vi "roboRIO Set Pin Info.vi"(7 "Size":i32=30, 9 "Pin Info Array":T2, 11 "Display State In in":T1 caption="State") -> (1 "Data":bool[](array[boolean]), 3 "Display State In out":T1 caption="State")   [LabVIEW 2021]
uses:
  <vilib>/myRIO/Common/Instrument Driver Framework/Utilities/xctls/utilities/typedefs/myRIOXC Pin Info Array.ctl
  <vilib>/myRIO/Common/Instrument Driver Framework/Utilities/xctls/utilities/typedefs/myRIOXC Pin Info.ctl
  <vilib>/myRIO/Common/Instrument Driver Framework/Utilities/xctls/utilities/typedefs/roboRIO Bank Display State.ctl
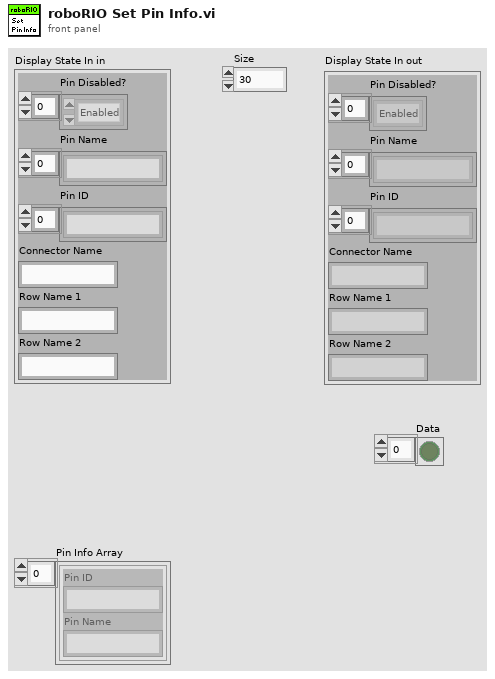
[diagram p1: front panel]
types:
  T1 = typedef "roboRIO Bank Display State.ctl" = cluster{"Pin Disabled?":enum8{"Enabled", "Disabled", "Disabled and Grayed Out"}[], "Pin Name":string[], "Pin ID":string[], "Connector Name":string, "Row Name 1":string, "Row Name 2":string}
  T2 = typedef "myRIOXC Pin Info Array.ctl" = T3[]
  T3 = typedef "myRIOXC Pin Info.ctl" = cluster{"Pin ID":string, "Pin Name":string}
  T4 = enum8{"Enabled", "Disabled", "Disabled and Grayed Out"}
  T5 = enum8{"Enabled", "Disabled", "Disabled and Grayed Out"}[]
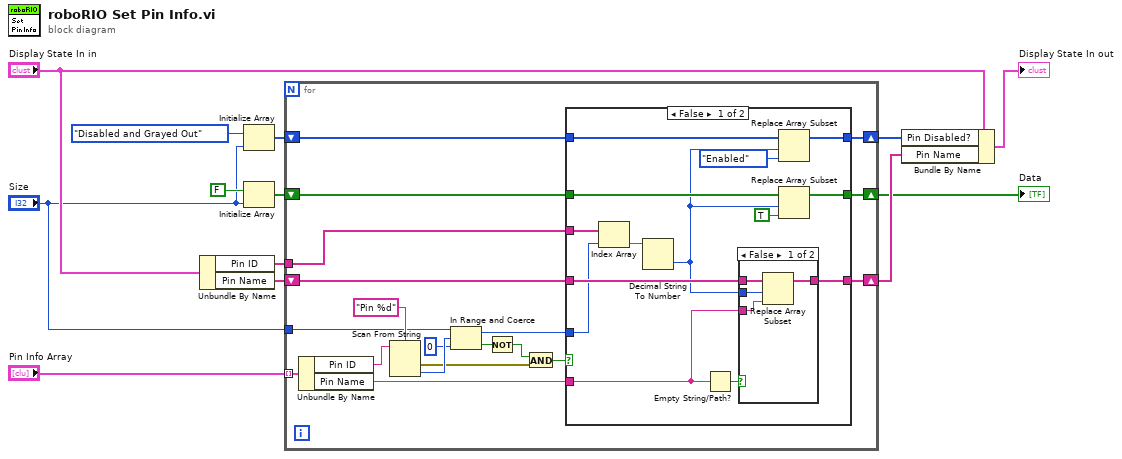
[diagram p0: block diagram]
diagram:
  n1 = Unbundle By Name("Display State In in") -> ("Pin ID"=w2:string[], "Pin Name"=w5:string[])
  n2 = Initialize Array(T4."Disabled and Grayed Out" ("Disabled"), "Size") -> (w3:T5)
  n3 = Initialize Array(FALSE, "Size") -> (w6:bool[])
  n4 = for {
    tunnel: "Pin Info Array" -> [w32] mode=indexing
    shift-right: [w31] -> w12
    shift-left: w3 -> [w30]
    shift-right: [w29] -> w13
    shift-left: w5 -> [w28]
    shift-right: [w25] -> w8
    shift-left: w6 -> [w26]
    tunnel: w2 -> [w22]
    tunnel: "Size" -> [w20]
    n5 = Unbundle By Name(w32) -> ("Pin ID"=w24:string, "Pin Name"=w27:string)
    n6 = Scan From String(format string="Pin %d", input string=w24) -> (error out=w16:errorcluster, output 1=w21:i32)  [unwired: 3 in, 2 out]
    n7 = In Range and Coerce(upper limit=w20, x=w21, lower limit=0) -> (coerced(x)=w18:i32, In Range?=w17:bool)
    n8 = Not(x=w17) -> (.not. x?=w15:bool)
    n9 = And(x=w15, y=w16) -> (x .and. y?=w14:bool)
    n10 = case shown="False" w14 {
      tunnel: [w46 w52] -> w31
      tunnel: w30 -> [w45 w52]
      tunnel: [w44 w54] -> w29
      tunnel: w28 -> [w39 w54]
      tunnel: w27 -> [w37 _]
      tunnel: w26 -> [w42 w53]
      tunnel: [w41 w53] -> w25
      tunnel: w18 -> [w35 _]
      tunnel: w22 -> [w36 _]
      frame False {
        n11 = Index Array(array=w36, index=w35) -> (element=w34:string)
        n12 = Decimal String To Number(string=w34) -> (number=w33:i32)  [unwired: 2 in, 1 out]
        n13 = Empty String/Path?(string/path=w37) -> (empty?=w40:bool)
        n14 = case shown="False" w40 {
          tunnel: [w50 w51] -> w44
          tunnel: w39 -> [w49 w51]
          tunnel: w33 -> [w48 _]
          tunnel: w37 -> [w47 _]
          frame False {
            n15 = Replace Array Subset(array=w49, new element=w47, index=w48) -> (w50:string[])
          }
          frame True {
          }
        }
        n16 = Replace Array Subset(array=w45, new element=T4."Enabled" ("Disabled"), index=w33) -> (w46:T5)
        n17 = Replace Array Subset(array=w42, new element=TRUE ("new element/subarray"), index=w33) -> (w41:bool[])
      }
      frame True {
      }
    }
  }
  "Data" <- w8
  n18 = Bundle By Name(cluster="Display State In in", "Pin Disabled?"=w12, "Pin Name"=w13) -> (→"Display State In out":T1)
